vi "sendData.vi"(8 "error in (no error)":errorcluster, 11 "StepperMotor in":refnum<class "StepperMotor.lvclass">) -> (0 "error out":errorcluster, 3 "StepperMotor out":refnum<class "StepperMotor.lvclass">)   [LabVIEW 2013, in "StepperMotor.lvclass"]
uses:
  StepperMotor.lvclass
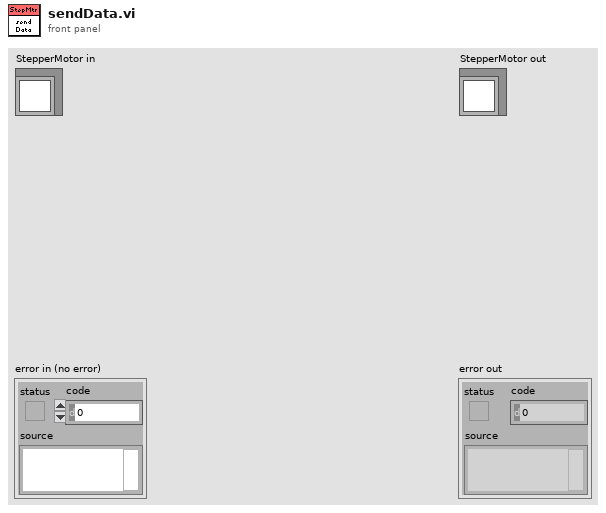
[diagram p1: front panel]
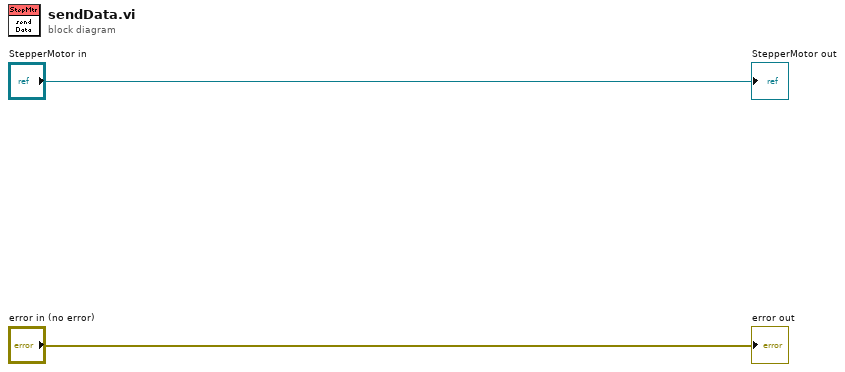
[diagram p0: block diagram]
diagram:
  "error out" <- "error in (no error)"
  "StepperMotor out" <- "StepperMotor in"
